vi "mediaIntesecaoCameras.vi"() -> ()   [LabVIEW 2018]
uses:
  <vilib>/Analysis/Matrix/Datatypes/RealMatrix.ctl
  <vilib>/Analysis/Matrix/NI_Matrix.lvlib
  SSL Detection Robot.ctl
  SSL Detection Ball.ctl
  SSL Detection Frame.ctl
panel:
  out "output cluster":T1 {"robots_blue"."height" format="%+4.3f"; "robots_blue"."pixel_y" format="%+4.3f"; "robots_blue"."pixel_x" format="%+4.3f"; "robots_blue"."orientation" format="%+4.3f"; "robots_blue"."y" format="%+4.3f"; "robots_blue"."confidence" format="%4.3f"; "robots_blue"."x" format="%+4.3f"; "robots_yellow"."height" format="%+4.3f"; "robots_yellow"."pixel_y" format="%+4.3f"; "robots_yellow"."pixel_x" format="%+4.3f"; "robots_yellow"."orientation" format="%+4.3f"; "robots_yellow"."y" format="%+4.3f"; "robots_yellow"."confidence" format="%4.3f"; "robots_yellow"."x" format="%+4.3f"}
  in  "Field Size 2":T5
  in  "Array":T1[](array[typedef]) {"robots_blue"."height" format="%+4.3f"; "robots_blue"."pixel_y" format="%+4.3f"; "robots_blue"."pixel_x" format="%+4.3f"; "robots_blue"."orientation" format="%+4.3f"; "robots_blue"."y" format="%+4.3f"; "robots_blue"."confidence" format="%4.3f"; "robots_blue"."x" format="%+4.3f"; "robots_yellow"."height" format="%+4.3f"; "robots_yellow"."pixel_y" format="%+4.3f"; "robots_yellow"."pixel_x" format="%+4.3f"; "robots_yellow"."orientation" format="%+4.3f"; "robots_yellow"."y" format="%+4.3f"; "robots_yellow"."confidence" format="%4.3f"; "robots_yellow"."x" format="%+4.3f"}
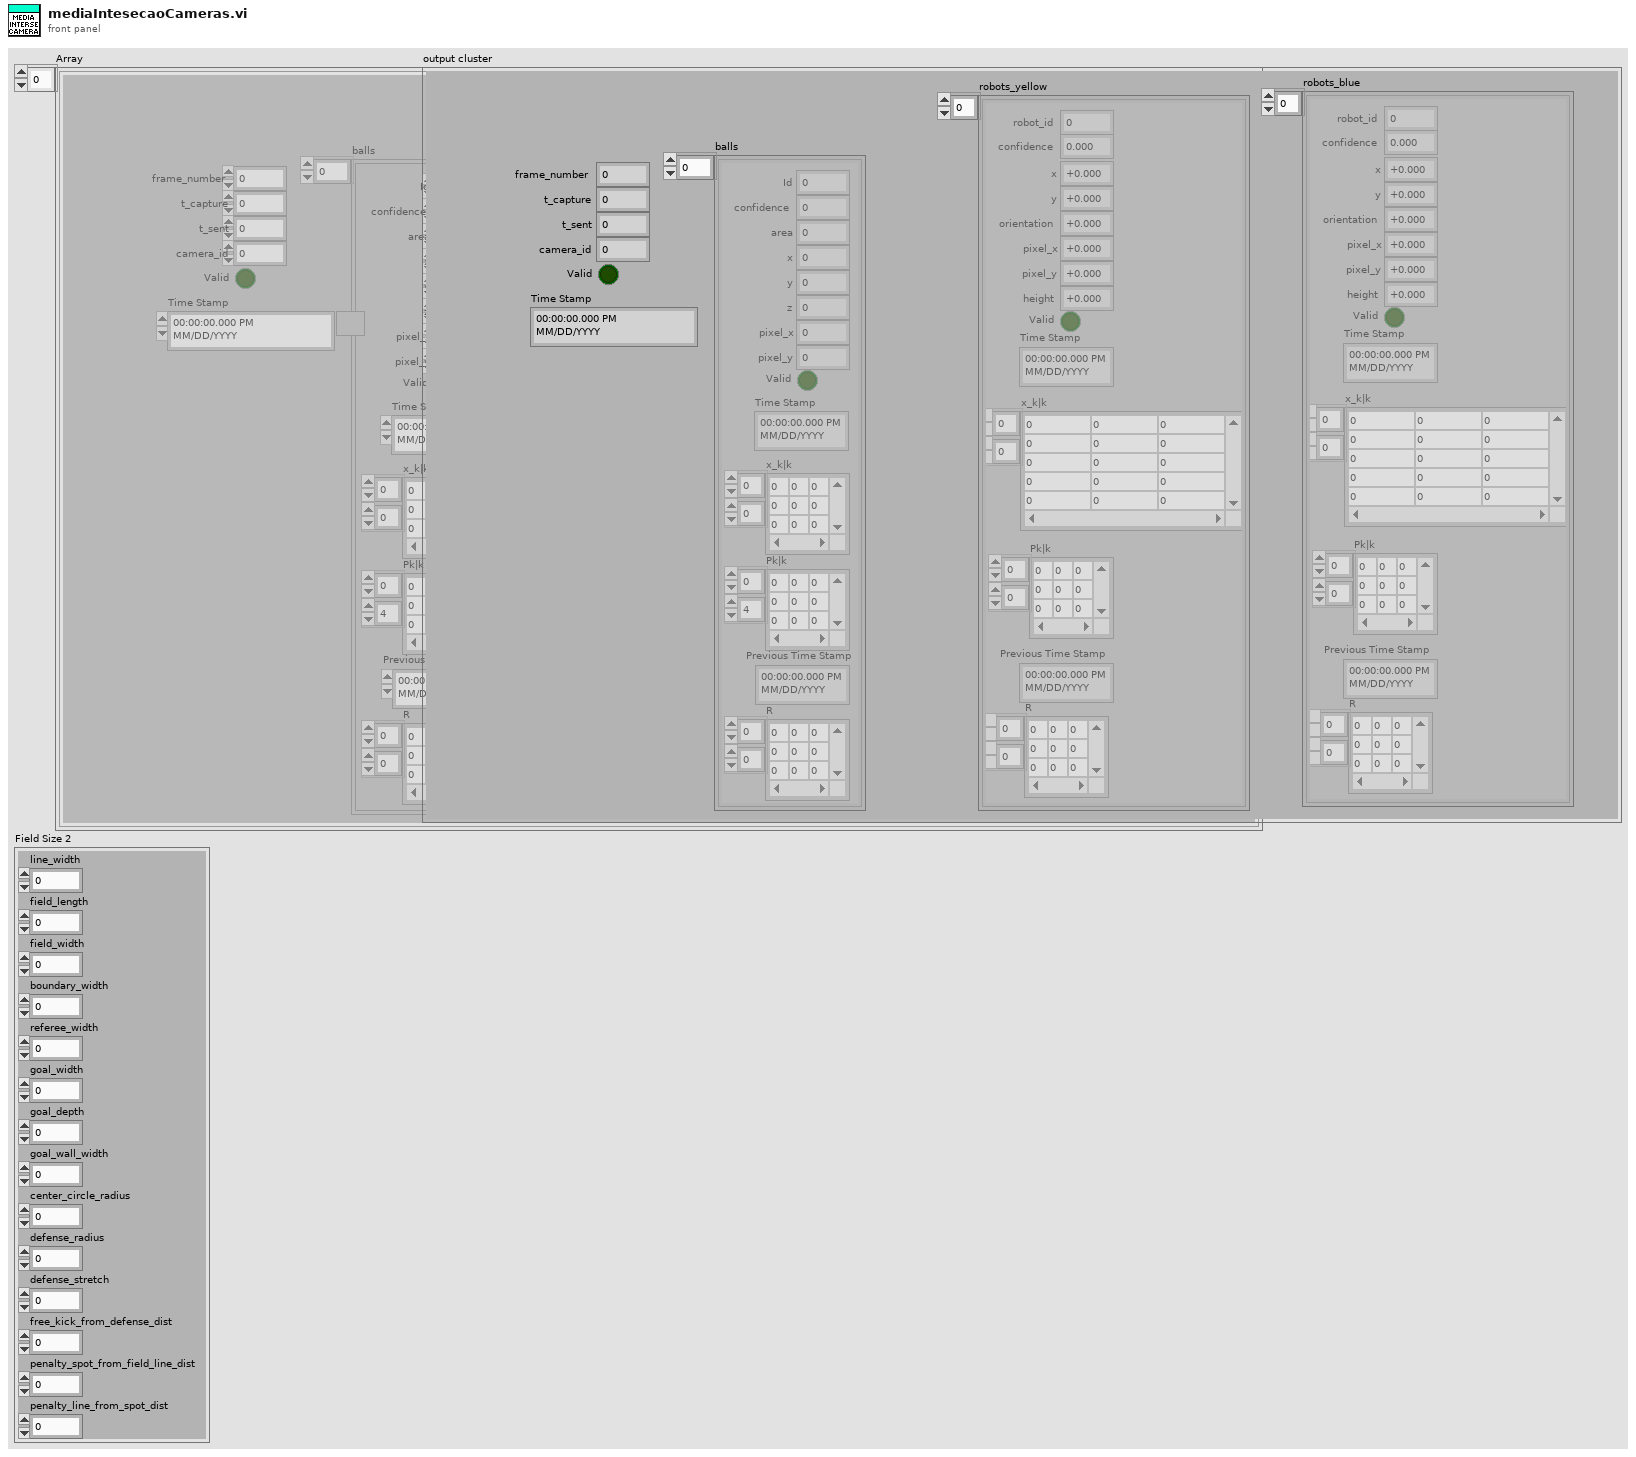
[diagram p1: front panel]
types:
  T1 = typedef "SSL Detection Frame.ctl" = cluster{"frame_number":u32, "t_capture":dbl, "t_sent":dbl, "camera_id":u32, "robots_yellow":T2[], "robots_blue":T2[], "balls":T4[], "Valid":bool, "Time Stamp":timestamp}
  T2 = typedef "SSL Detection Robot.ctl" = cluster{"x":sgl, "robot_id":u32, "confidence":sgl, "y":sgl, "orientation":sgl, "pixel_x":sgl, "pixel_y":sgl, "height":sgl, "Valid":bool, "Time Stamp":timestamp, "x_k|k":T3, "Pk|k":T3, "Previous Time Stamp":timestamp, "R":T3}
  T3 = typedef "NI_Matrix.lvlib/RealMatrix.ctl" = dbl[][]
  T4 = typedef "SSL Detection Ball.ctl" = cluster{"x":sgl, "area":u32, "confidence":sgl, "y":sgl, "z":sgl, "pixel_x":sgl, "pixel_y":sgl, "Valid":bool, "Time Stamp":timestamp, "x_k|k":T3, "Pk|k":T3, "Id":u32, "Previous Time Stamp":timestamp, "R":T3}
  T5 = cluster{"line_width":u32, "field_length":u32, "field_width":u32, "boundary_width":u32, "referee_width":u32, "goal_width":u32, "goal_depth":u32, "goal_wall_width":u32, "center_circle_radius":u32, "defense_radius":u32, "defense_stretch":u32, "free_kick_from_defense_dist":u32, "penalty_spot_from_field_line_dist":u32, "penalty_line_from_spot_dist":u32}
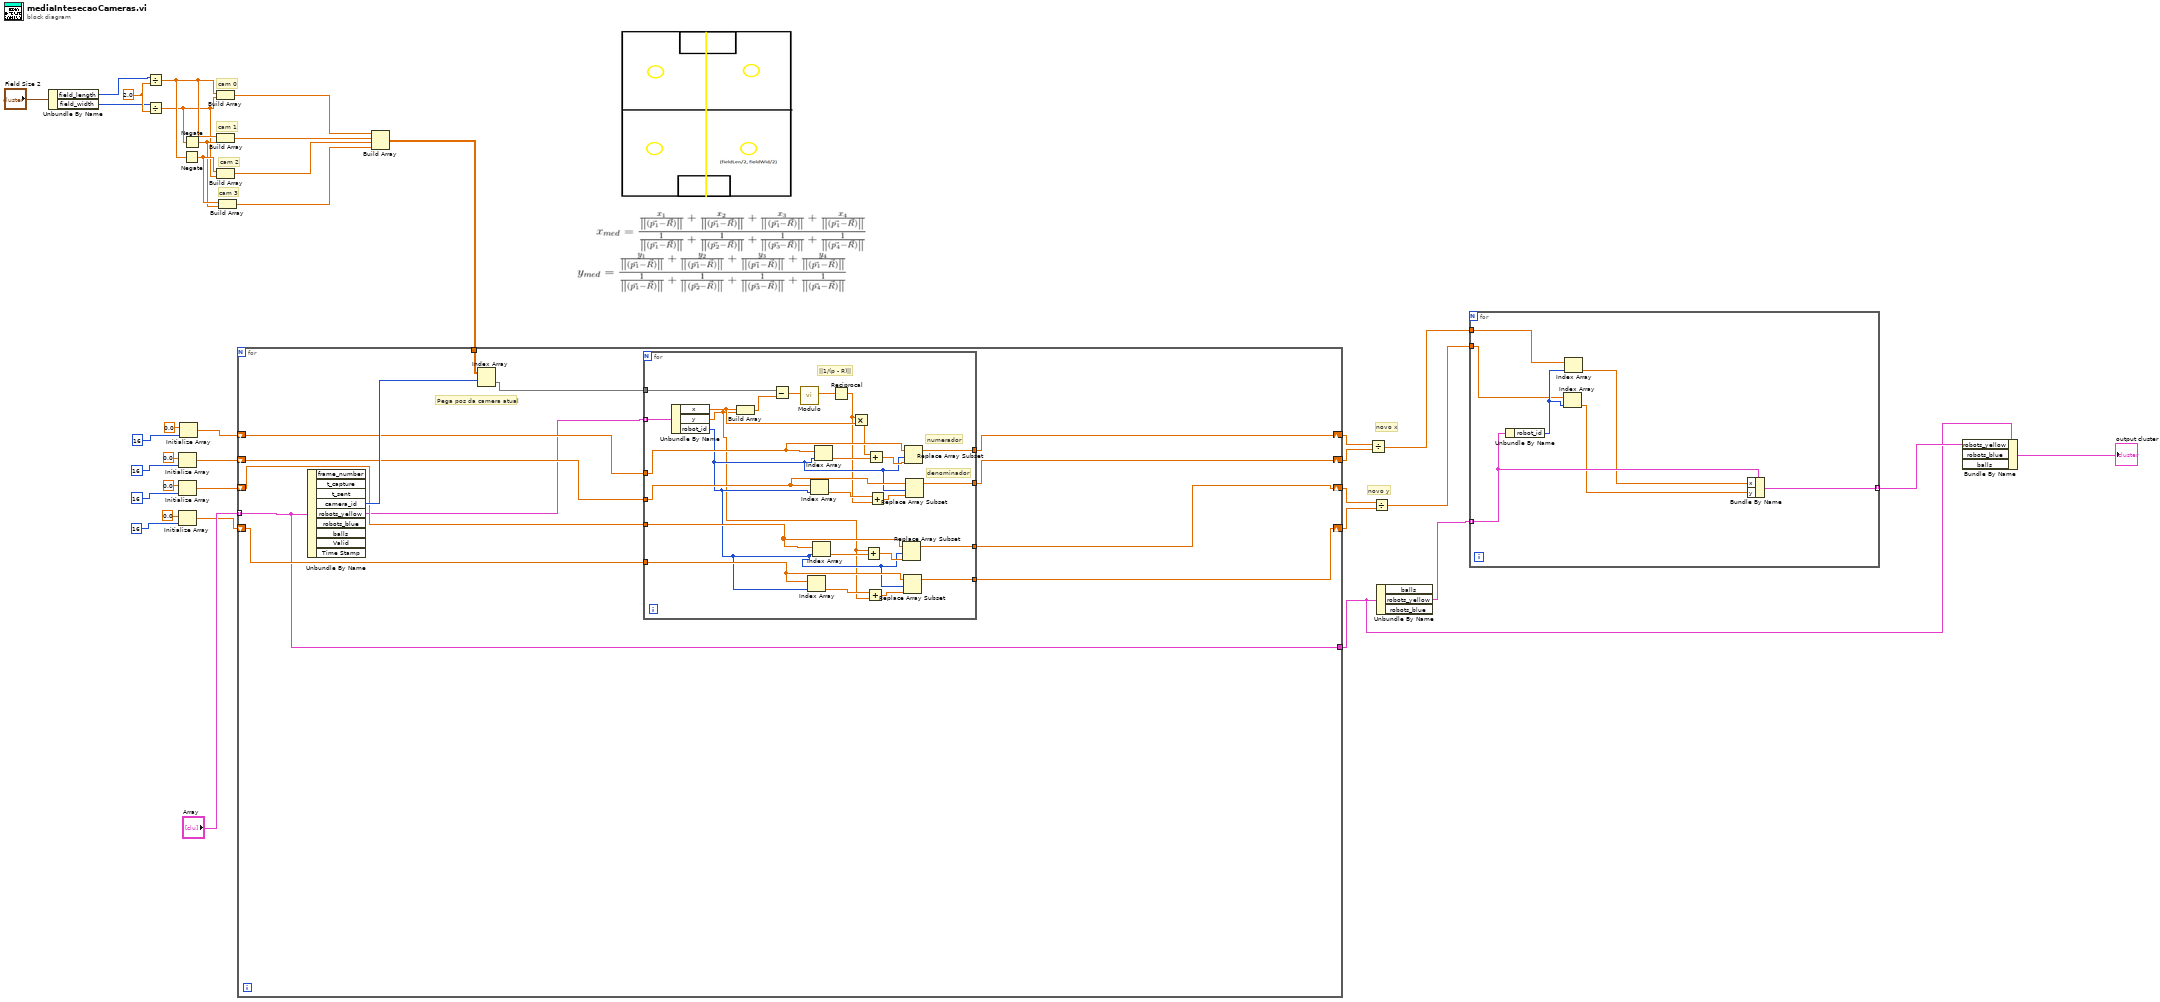
[diagram p0: block diagram]
diagram:
  w34 = 2.0 ("y")
  # "novo y"
  # "novo x"
  # "cam 3"
  # "cam 2"
  # "cam 1"
  # "cam 0"
  n1 = Unbundle By Name("Field Size 2") -> ("field_length"=w33:u32, "field_width"=w32:u32)
  n2 = Divide(x=w33, y=w34) -> (x/y=w30:dbl)
  n3 = Divide(x=w32, y=w34) -> (x/y=w28:dbl)
  n4 = Initialize Array(0.0 ("element"), 16 ("dimension size")) -> (w11:dbl[])
  n5 = Initialize Array(0.0 ("element"), 16 ("dimension size")) -> (w17:dbl[])
  n6 = Initialize Array(0.0 ("element"), 16 ("dimension size")) -> (w12:dbl[])
  n7 = Initialize Array(0.0 ("element"), 16 ("dimension size")) -> (w20:dbl[])
  n8 = Negate(x=w30) -> (-x=w31:dbl)
  n9 = Negate(x=w28) -> (-x=w29:dbl)
  n10 = Build Array(w30, w28) -> (w27:dbl[])
  n11 = Build Array(w30, w29) -> (w26:dbl[])
  n12 = Build Array(w31, w28) -> (w25:dbl[])
  n13 = Build Array(w31, w29) -> (w24:dbl[])
  n14 = Build Array(w27, w26, w25, w24) -> (w23:dbl[][])
  n15 = for {
    tunnel: "Array" -> [w37] mode=indexing
    tunnel: w23 -> [w49]
    shift-right: [w44] -> w10
    shift-left: w20 -> [w46]
    shift-right: [w43] -> w9
    shift-left: w17 -> [w45]
    shift-right: [w40] -> w8
    shift-left: w12 -> [w42]
    shift-right: [w39] -> w7
    shift-left: w11 -> [w41]
    tunnel: [w37] -> w1
    # "Pega pos da camera atual"
    n16 = Unbundle By Name(w37) -> ("camera_id"=w48:u32, "robots_yellow"=w38:T2[])  [unwired: 7 out]
    n17 = Index Array(array=w49, index (row)=w48) -> (element=w47:dbl[])  [unwired: 1 in]
    n18 = for {
      tunnel: w38 -> [w75] mode=indexing
      tunnel: w47 -> [w73]
      tunnel: w46 -> [w67]
      tunnel: w45 -> [w63]
      tunnel: [w69] -> w44
      tunnel: [w68] -> w43
      tunnel: w42 -> [w56]
      tunnel: w41 -> [w55]
      tunnel: [w52] -> w40
      tunnel: [w51] -> w39
      # "denominador"
      # "numerador"
      # "||1/(p - R)||"
      n19 = Unbundle By Name(w75) -> ("x"=w70:sgl, "y"=w50:sgl, "robot_id"=w54:u32)
      n20 = Build Array(w70, w50) -> (w74:sgl[])
      n21 = Subtract(x=w73, y=w74) -> (x-y=w72:dbl[])
      n22 = call "Modulo.vi"("2D vector"=w72) -> ("Modulo"=w71:dbl)  [unwired: 10 in]
      n23 = Index Array(array=w55, index=w54) -> (element=w58:dbl)
      n24 = Index Array(array=w63, index=w54) -> (element=w62:dbl)
      n25 = Index Array(array=w56, index=w54) -> (element=w60:dbl)
      n26 = Index Array(array=w67, index=w54) -> (element=w65:dbl)
      n27 = Reciprocal(x=w71) -> (1/x=w53:dbl)
      n28 = Multiply(x=w53, y=w70) -> (x*y=w66:dbl)
      n29 = Add(x=w50, y=w60) -> (x+y=w59:dbl)
      n30 = Add(x=w58, y=w50) -> (x+y=w57:dbl)
      n31 = Add(x=w66, y=w65) -> (x+y=w64:dbl)
      n32 = Add(x=w62, y=w53) -> (x+y=w61:dbl)
      n33 = Replace Array Subset(array=w56, new element=w59, index=w54) -> (w52:dbl[])
      n34 = Replace Array Subset(array=w55, new element=w57, index=w54) -> (w51:dbl[])
      n35 = Replace Array Subset(array=w67, new element=w64, index=w54) -> (w69:dbl[])
      n36 = Replace Array Subset(array=w63, new element=w61, index=w54) -> (w68:dbl[])
    }
  }
  n37 = Divide(x=w10, y=w9) -> (x/y=w6:dbl[])
  n38 = Divide(x=w8, y=w7) -> (x/y=w5:dbl[])
  n39 = Unbundle By Name(w1) -> ("robots_yellow"=w4:T2[])  [unwired: 2 out]
  n40 = for {
    tunnel: w6 -> [w81]
    tunnel: w5 -> [w79]
    tunnel: w4 -> [w82] mode=indexing
    tunnel: [w76] -> w3 mode=indexing
    n41 = Unbundle By Name(w82) -> ("robot_id"=w80:u32)
    n42 = Index Array(array=w79, index=w80) -> (element=w77:dbl)
    n43 = Index Array(array=w81, index=w80) -> (element=w78:dbl)
    n44 = Bundle By Name(cluster=w82, "x"=w78, "y"=w77) -> (w76:T2)
  }
  n45 = Bundle By Name(cluster=w1, "robots_yellow"=w3) -> (→"output cluster":T1)  [unwired: 2 in]
